vi "Test Set, Record Results.vi"(7 "step name (\"\")":string, 8 "error in":errorcluster, 9 "test case":string="DriveC", 10 "Result":dbl=nan format="%.3g", 11 "Sequence Context":refnum<k7>) -> (0 "error out":errorcluster, 3 "Sequence Context dup":refnum<k7>)   [LabVIEW 2010]
doc: "This function transfers a single Compare Data Test (CDT) record to the current TestStand sequence step."
uses:
  Generic/TestConsole/Test Criteria Control.ctl
panel:
  in  "Acceptance Criteria":T1
  in  "Test Criteria":T1=[["TRS1553", "Drive C: Free Space", "", "2.00", "", "GB", "GT", "%.2f", "%.2f", "DriveC"], ["TRS1553", "Drive D: Free Space", "", "2.00", "", "GB", "GT", "%.2f", "%.2f", "DriveD"], ["TRS1554", "Free Memory", "", "50.0", "", "%", "GT", "%.2f", "%.2f", "FreeMem"], ["", "DIG1 Ch1&2 Mean DC Offset", "", "-5.000", "5.000", "mV", "GELE", "%.3f", "%.3f", "Offset"]]
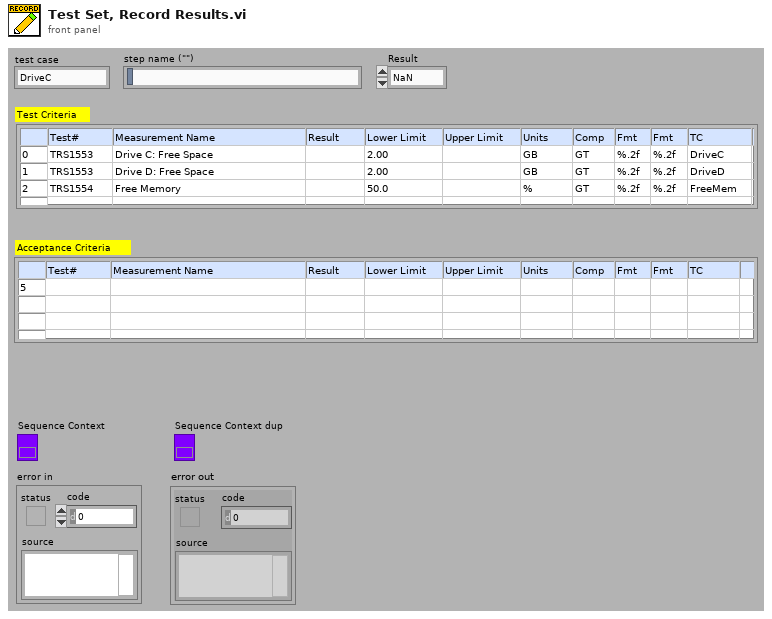
[diagram p1: front panel]
types:
  T1 = typedef "Test Criteria Control.ctl" = string[][]
  T2 = typedef "TestStand_Result Control.ctl" = cluster{"Measurement Name":string, "Result":dbl, "Low Limit":dbl, "High Limit":dbl, "Units":string, "Comp":string, "DataFmt":string, "LimitFmt":string}
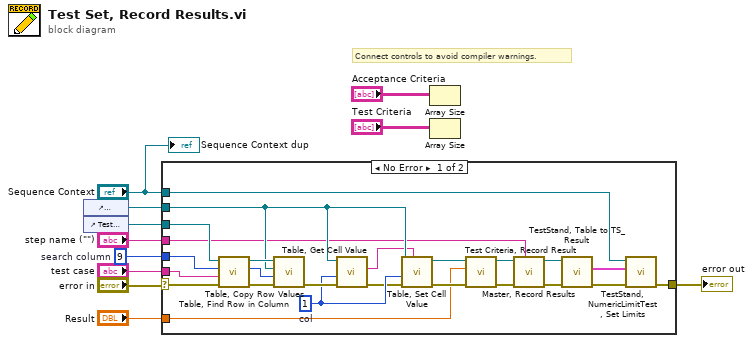
[diagram p0: block diagram]
diagram:
  w2 = 9  # search column
  # "Connect controls to avoid compiler warnings."
  n1 = control-ref of="Acceptance Criteria"() -> (w4:refnum<vi>)
  n2 = control-ref of="Test Criteria"() -> (w6:refnum<vi>)
  n3 = case shown="No Error" "error in" {
    selector: "error in" -> [w16 w36]
    tunnel: [w27 w36] -> w11
    tunnel: "Sequence Context" -> [w34 _]
    tunnel: "test case" -> [w15 _]
    tunnel: w6 -> [w35 _]
    tunnel: w4 -> [w19 _]
    tunnel: "Result" -> [w28 _]
    tunnel: w2 -> [w26 _]
    tunnel: "step name (\"\")" -> [w13 _]
    frame No Error {
      w18 = 1  # col
      n4 = call "Table, Find Row in Column.vi"("error in"=w16, "search key"=w15, "search column (0)"=w26, "Tbl Refnum"=w35) -> ("error out"=w33:errorcluster, "row index"=w31:i32, "Tbl Refnum out"=w32:refnum<vi>)  [unwired: 4 in, 1 out]
      n5 = call "Table, Copy Row Values.vi"("error in"=w33, "row (0)"=w31, "Tbl Refnum Dst"=w19, "Tbl Refnum Src"=w32) -> ("error out"=w20:errorcluster)  [unwired: 3 in, 2 out]
      n6 = call "Table, Get Cell Value.vi"("error in"=w20, "column (0)"=w18, "Tbl Refnum"=w19) -> ("error out"=w14:errorcluster, "cell value"=w12:string)  [unwired: 6 in, 1 out]
      n7 = call "Table, Set Cell Value.vi"("cell value"=w12, "error in"=w14, "column (0)"=w18, "Tbl Refnum"=w19) -> ("error out"=w30:errorcluster, "Tbl Refnum out"=w29:refnum<vi>)  [unwired: 2 in, 2 out]
      n8 = call "Test Criteria, Record Result.vi"("error in"=w30, "Result"=w28, "Tbl Refnum"=w29) -> ("error out"=w25:errorcluster, "Tbl Refnum out"=w24:refnum<vi>)  [unwired: 6 in, 1 out]
      n9 = call "Master, Record Results.vi"("step name"=w13, "error in"=w25, "Tbl Refnum"=w24) -> ("error out"=w23:errorcluster, "Tbl Refnum dup"=w21:refnum<vi>)  [unwired: 7 in]
      n10 = call "TestStand, Table to TS_Result.vi"("error in"=w23, "Tbl Refnum"=w21) -> ("error out"=w22:errorcluster, "TestStand Result"=w17:T2)  [unwired: 7 in, 1 out]
      n11 = call "TestStand, NumericLimitTest, Set Limits.vi"("error in"=w22, "CDT_type"=w17, "Sequence Context"=w34) -> ("error out"=w27:errorcluster)  [unwired: 7 in, 1 out]
    }
    frame Error {
    }
  }
  "error out" <- w11
  n12 = Array Size(array="Acceptance Criteria") -> ()  [unwired: 1 out]
  n13 = Array Size(array="Test Criteria") -> ()  [unwired: 1 out]
  "Sequence Context dup" <- "Sequence Context"
